vi "Target Yaw Crossover.vi"(10 "Yaw in":dbl, 11 "Adjustment":dbl) -> (3 "Numeric out":dbl)   [LabVIEW 2018]
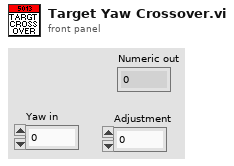
[diagram p1: front panel]
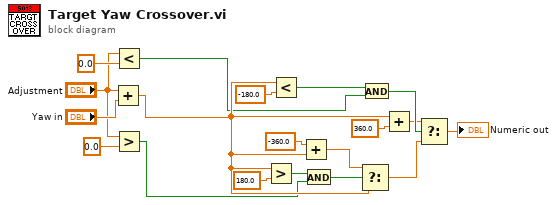
[diagram p0: block diagram]
diagram:
  n1 = Add(x="Adjustment", y="Yaw in") -> (x+y=w6:dbl)
  n2 = Less?(x="Adjustment", y=0.0 ("Y-Axis")) -> (x < y?=w1:bool)
  n3 = Greater?(x="Adjustment", y=0.0 ("Y-Axis")) -> (0:w2:bool)
  n4 = Greater?(x=w6, y=180.0) -> (0:w13:bool)
  n5 = Less?(x=w6, y=-180.0) -> (x < y?=w18:bool)
  n6 = Add(x=-360.0, y=w6) -> (x+y=w10:dbl)
  n7 = And(x=w13, y=w2) -> (x .and. y?=w12:bool)
  n8 = Select(t=w10, s=w12, f=w6) -> (s? t:f=w9:dbl)
  n9 = And(x=w18, y=w1) -> (x .and. y?=w17:bool)
  n10 = Add(x=w6, y=360.0) -> (x+y=w15:dbl)
  n11 = Select(t=w15, s=w17, f=w9) -> (s? t:f=→"Numeric out":dbl)
